vi "set dt.vi"(10 "dt":u32=1, 11 "timing source in":refnum<class "TBM timing source.lvclass">) -> (3 "timing source out":refnum<class "TBM timing source.lvclass">)   [LabVIEW 2013, in "TBM timing source.lvclass"]
doc: "Sets the value of <b>dt</b> which is the number of ticks of the desired clock which should elapse between iterations. This behavior is generally the same as the behavior of the timed loop."
uses:
  TBM timing source.lvclass
  TBM timing source.lvclass/TBM timing source.ctl
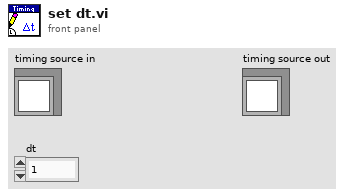
[diagram p1: front panel]
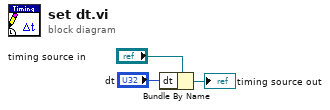
[diagram p0: block diagram]
diagram:
  n1 = Bundle By Name(cluster="timing source in", "dt"="dt") -> (→"timing source out":refnum<class "TBM timing source.lvclass">)
